vi "UDSWrapper.vi"(0 "UDS Action":T4, 1 "Session Type":u16(ring) items=["Default Session"=1, "ECU Programming Session"=2, "ECU Extended Diagnostic Session"=3], 2 "Reset Mode":u16(ring) items=["Hard Reset"=1, "Key Off On Reset"=2, "Soft Reset"=3, "Enable Rapid Power Shutdown "=4, "Disable Rapid Power Shutdown"=5], 3 "SessionID":string, 5 "UDS Session Parameters":T1={"XNET Interface"="CAN1@nixnet", "BaudRate"=500000, "Transmit ID"=470077443, "Receive ID"=470073347} {"Receive ID" format="%x"; "Transmit ID" format="%x"}, 7 "Tester Present":T3={"Start Tester Present"=FALSE, "Tester Present Period"=1.0}, 9 "ID":u16 format="%.0x", 11 "error in (no error)":errorcluster, 12 "Byte Data To Write":u8[](array[numeric]) format="%.0x", 13 "String Data To Write":string) -> (6 "Success ?":bool, 8 "Read Data":T2, 15 "error out":errorcluster)   [LabVIEW 2021, in "Lunar UDS CAN.lvlib"]
uses:
  Lunar UDS CAN.lvlib
  Controls/UDSActions.ctl
  Controls/UDSReadData.ctl
  Controls/UDSSessionParameters.ctl
  <vilib>/Automotive Diagnostic Command Set/Diagnostic Transport.llb/Diag Reference.ctl
  <vilib>/Automotive Diagnostic Command Set/Diagnostic Transport.llb/Transport Protocol Selector.ctl
  <vilib>/Automotive Diagnostic Command Set/Diagnostic Transport.llb/DoIP Protocol Version.ctl
  <vilib>/Automotive Diagnostic Command Set/Diagnostic Transport.llb/Diag Globals.ctl
  <vilib>/addons/Automotive Diagnostic Command Set/NI_Automotive Diagnostic Command Set.lvlib
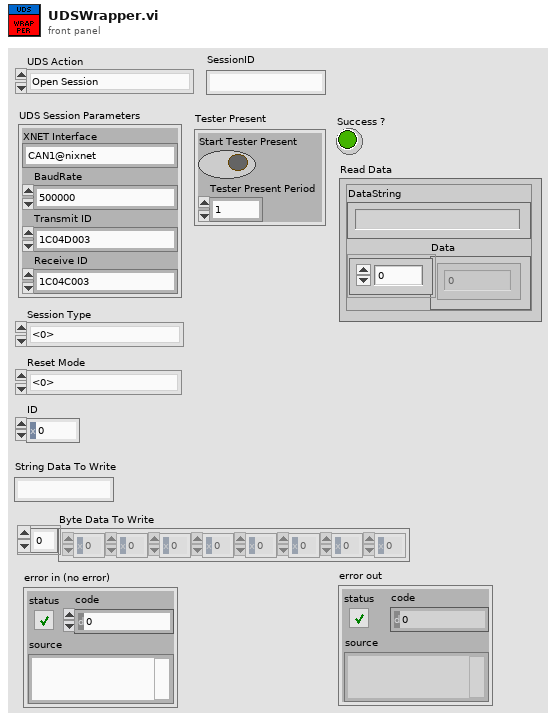
[diagram p1: front panel]
types:
  T1 = typedef "Lunar UDS CAN.lvlib/UDSSessionParameters.ctl" = cluster{"XNET Interface":string, "BaudRate":u64, "Transmit ID":i32, "Receive ID":i32}
  T2 = typedef "Lunar UDS CAN.lvlib/UDSReadData.ctl" = cluster{"DataString":string, "Data":i32[]}
  T3 = cluster{"Start Tester Present":bool, "Tester Present Period":dbl}
  T4 = typedef "Lunar UDS CAN.lvlib/UDSActions.ctl" = enum16{"Open Session", "Connect To Diagnostic Session", "Send Tester Present", "ECU Reset", "Write String Data", "Write Byte Data", "Read Data", "Close Session", "Close All Sessions"}
  T5 = typedef "NI_Automotive Diagnostic Command Set.lvlib/Diag Reference.ctl" = cluster{"Diag CAN Handle":u32, "Transport Protocol":T6, "Receive Address Extension":u8, "Transmit Address Extension":u8, "Receive CAN Id":u32, "Transmit CAN Id":u32, "Log Frames ?":bool, "My TP Address":u8, "Other TP Address":u8, "T1":u16, "T2":u16, "T3":u16, "T4":u16, "Tx SN":u8, "Block Size":u8, "Rx SN":u8, "VW TP Initialized?":bool, "Tx block no":u8, "baud rate":u64, "Interface":string, "Channel Diag CAN Handle":u32, "UDP Connection ID":refnum<k16>, "TCP Connection ID":refnum<k5>, "Target IP Addr":u32, "Source Address":u16, "Target Address":u16, "Send Header NACK?":bool, "DLL Handle":u32, "NAD":u8, "Time Stamp read first":dbl, "Time Stamp read last":dbl, "Time Stamp write first":dbl, "Time Stamp write last":dbl, "Time Stamp write":dbl, "Time Stamp read":dbl, " I/O Mode":u32, "FD Baudrate":u64, "TX_DL":u16, "RX_DL":u16, "DoIP Protocol Version":T7, " Selected I/O Mode":u32, "TesterPresent Counter":u32, "TesterPresent Limit":u32, "TesterPresent Tick[ms]":i32, "TesterPresent RequireResponse?":bool, "TesterPresent Stored Ref?":bool, "TesterPresent Message":u8[], "TesterPresent Task Handle":i32, "TesterPresent Semaphore":T8, "Response Plausibility Check":u32, "Default Version?":bool, "Diagostic Globals":T9, "Session-based Properties?":bool, "NI-XNET IP Stack Reference":i64, "NI-XNET IP Stack TCP Reference":i64, "NI-XNET IP Stack UDP Reference":i64, "NI-XNET IP Stack Local Interface":string, "Functional CAN Id":u32, "Diag CAN Queue":refnum<queue>, "Frame Fillling Mode":u32, "DoIP Acknowledge Mode":u32, "Message Buffer":u8[]}
  T6 = typedef "NI_Automotive Diagnostic Command Set.lvlib/Transport Protocol Selector.ctl" = enum16{"ISO TP - Normal Mode", "ISO TP - Mixed Mode", "VW TP 2.0", "Diagnostics on IP", "ISO TP LIN"}
  T7 = typedef "NI_Automotive Diagnostic Command Set.lvlib/DoIP Protocol Version.ctl" = u8
  T8 = typedef "Semaphore RefNum" = refnum<k1>
  T9 = typedef "NI_Automotive Diagnostic Command Set.lvlib/Diag Globals.ctl" = cluster{"Timeout FC (Bs)":u32, "Timeout CF (Cr)":u32, "Timeout Diag Command":u32, "Receive Block Size (BS)":u8, "Wait Time CF (STmin)":u8, "Max Waits (N_WFTmax)":u8, "Waits to Send (N_WAIT)":i32, "Time between Waits (TW)":u32, "Fill CAN Frames?":bool, "Fill Byte":u32, "Invalid Response as Error?":bool, "Max RspPending Count":u32, "VWTP Command Timeout":u32, "Transport Protocol":T6, "Diag CAN Handle":u32, "DLL Handle":u32, "Timeout RspPending":u32}
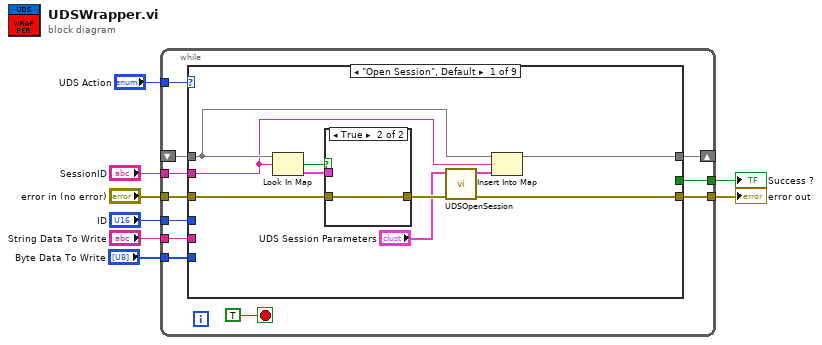
[diagram p0: block diagram]
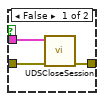
[diagram p2: hidden frame]
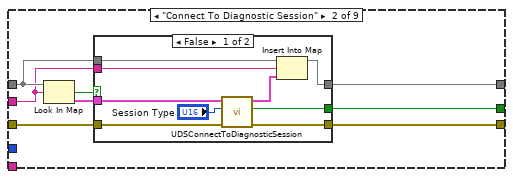
[diagram p3: hidden frame]
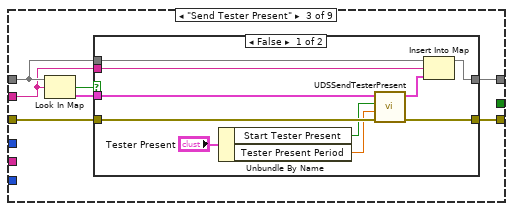
[diagram p5: hidden frame]
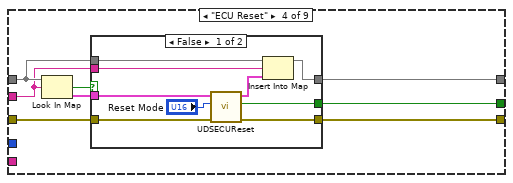
[diagram p7: hidden frame]
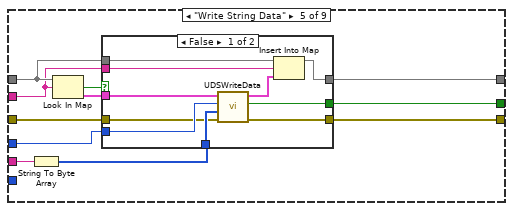
[diagram p9: hidden frame]
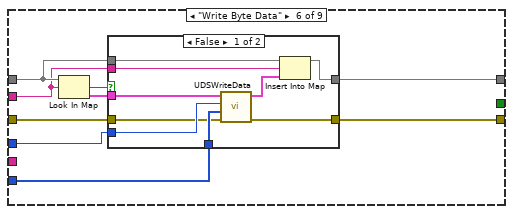
[diagram p11: hidden frame]
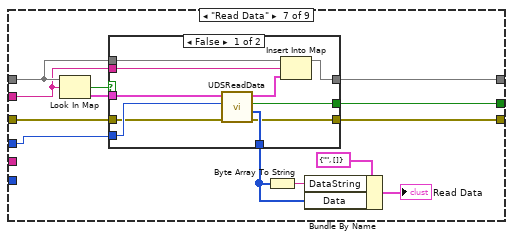
[diagram p13: hidden frame]
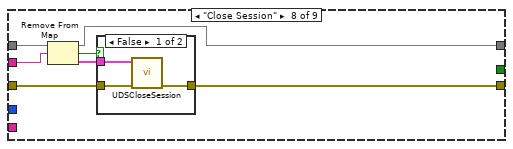
[diagram p15: hidden frame]
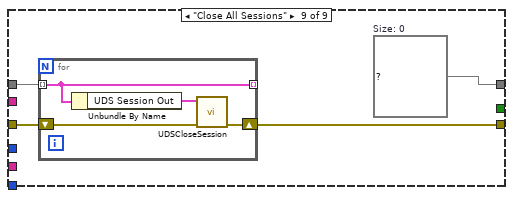
[diagram p17: hidden frame]
diagram:
  n1 = while {
    tunnel: "UDS Action" -> [w18]
    tunnel: "error in (no error)" -> [w17]
    tunnel: [w16] -> w6
    tunnel: [w15] -> w5
    tunnel: "ID" -> [w14]
    tunnel: "Byte Data To Write" -> [w13]
    tunnel: "String Data To Write" -> [w12]
    tunnel: "SessionID" -> [w11]
    shift-right: [w9] -> _
    shift-left: _ -> [w10]
    stop <- TRUE stop-if-true
    n2 = case shown="\"Open Session\", Default" w18 {
      tunnel: w17 -> [w26 w39 w57 w77 w98 w120 w140 w163 w171]
      tunnel: [w29 w38 w53 w76 w97 w119 w141 w159 w170] -> w16
      tunnel: [_ w37 _ w73 w94 _ w134 _ _] -> w15
      tunnel: w14 -> [_ _ _ _ w95 w117 w139 _ _]
      tunnel: w13 -> [_ _ _ _ _ w118 _ _ _]
      tunnel: w12 -> [_ _ _ _ w101 _ _ _ _]
      tunnel: w11 -> [w22 w35 w55 w74 w92 w114 w136 w161 _]
      tunnel: w10 -> [w24 w36 w56 w75 w93 w115 w137 w162 w172]
      tunnel: [w21 w34 w54 w72 w91 w116 w135 w160 w173] -> w9
      frame "Open Session", Default {
        n3 = Look In Map(map=w24, key=w22) -> (key not found?=w28:bool, value=w27:T5)  [unwired: 1 in]
        n4 = case shown="True" w28 {
          tunnel: w27 -> [w32 _]
          tunnel: w26 -> [w31 w33]
          tunnel: [w30 w33] -> w25
          frame False {
            n5 = call "UDSCloseSession.vi"("error in (no error)"=w31, "UDS Session In"=w32) -> ("error out"=w30:errorcluster)  [unwired: 9 in]
          }
          frame True {
          }
        }
        n6 = call "UDSOpenSession.vi"("error in (no error)"=w25, "UDS Session Parameters"="UDS Session Parameters") -> ("error out"=w29:errorcluster, "UDS Session Out"=w23:T5)  [unwired: 8 in]
        n7 = Insert Into Map(map in=w24, key=w22, value=w23) -> (map out=w21:map{string, T5})  [unwired: 2 out]
      }
      frame "Connect To Diagnostic Session" {
        n8 = Look In Map(map=w36, key=w35) -> (key not found?=w41:bool, value=w40:T5)  [unwired: 1 in]
        n9 = case shown="False" w41 {
          tunnel: w40 -> [w47 _]
          tunnel: w39 -> [w50 w52]
          tunnel: [w49 w52] -> w38
          tunnel: [w48 _] -> w37
          tunnel: w36 -> [w44 w51]
          tunnel: w35 -> [w43 _]
          tunnel: [w42 w51] -> w34
          frame False {
            n10 = call "UDSConnectToDiagnosticSession.vi"("error in (no error)"=w50, "Session Type"="Session Type", "UDS Session In"=w47) -> ("error out"=w49:errorcluster, "Connection Success ?"=w48:bool, "UDS Session Out"=w45:T5)  [unwired: 6 in]
            n11 = Insert Into Map(map in=w44, key=w43, value=w45) -> (map out=w42:map{string, T5})  [unwired: 2 out]
          }
          frame True {
          }
        }
      }
      frame "Send Tester Present" {
        n12 = Look In Map(map=w56, key=w55) -> (key not found?=w59:bool, value=w58:T5)  [unwired: 1 in]
        n13 = case shown="False" w59 {
          tunnel: w58 -> [w62 _]
          tunnel: w57 -> [w64 w71]
          tunnel: [w65 w71] -> w53
          tunnel: w56 -> [w69 w70]
          tunnel: w55 -> [w68 _]
          tunnel: [w67 w70] -> w54
          frame False {
            n14 = Unbundle By Name("Tester Present") -> ("Start Tester Present"=w61:bool, "Tester Present Period"=w60:dbl)
            n15 = call "UDSSendTesterPresent.vi"("error in (no error)"=w64, "Period"=w60, "Start"=w61, "UDS Session In"=w62) -> ("error out"=w65:errorcluster, "UDS Session Out"=w66:T5)  [unwired: 6 in]
            n16 = Insert Into Map(map in=w69, key=w68, value=w66) -> (map out=w67:map{string, T5})  [unwired: 2 out]
          }
          frame True {
          }
        }
      }
      frame "ECU Reset" {
        n17 = Look In Map(map=w75, key=w74) -> (key not found?=w79:bool, value=w78:T5)  [unwired: 1 in]
        n18 = case shown="False" w79 {
          tunnel: w78 -> [w88 _]
          tunnel: w77 -> [w87 w90]
          tunnel: [w85 w90] -> w76
          tunnel: w75 -> [w83 w89]
          tunnel: w74 -> [w82 _]
          tunnel: [w81 _] -> w73
          tunnel: [w80 w89] -> w72
          frame False {
            n19 = call "UDSECUReset.vi"("error in (no error)"=w87, "Reset Mode"="Reset Mode", "UDS Session In"=w88) -> ("error out"=w85:errorcluster, "success?"=w81:bool, "UDS Session Out"=w84:T5)  [unwired: 6 in]
            n20 = Insert Into Map(map in=w83, key=w82, value=w84) -> (map out=w80:map{string, T5})  [unwired: 2 out]
          }
          frame True {
          }
        }
      }
      frame "Write String Data" {
        n21 = String To Byte Array(string=w101) -> (unsigned byte array=w96:u8[])
        n22 = Look In Map(map=w93, key=w92) -> (key not found?=w100:bool, value=w99:T5)  [unwired: 1 in]
        n23 = case shown="False" w100 {
          tunnel: w99 -> [w102 _]
          tunnel: w98 -> [w105 w113]
          tunnel: [w106 w113] -> w97
          tunnel: w93 -> [w111 w112]
          tunnel: w92 -> [w110 _]
          tunnel: [w109 w112] -> w91
          tunnel: w96 -> [w108 _]
          tunnel: w95 -> [w107 _]
          tunnel: [w104 _] -> w94
          frame False {
            n24 = call "UDSWriteData.vi"("error in (no error)"=w105, "Data To Write"=w108, "ID"=w107, "UDS Session In"=w102) -> ("error out"=w106:errorcluster, "success?"=w104:bool, "UDS Session Out"=w103:T5)  [unwired: 5 in]
            n25 = Insert Into Map(map in=w111, key=w110, value=w103) -> (map out=w109:map{string, T5})  [unwired: 2 out]
          }
          frame True {
          }
        }
      }
      frame "Write Byte Data" {
        n26 = Look In Map(map=w115, key=w114) -> (key not found?=w122:bool, value=w121:T5)  [unwired: 1 in]
        n27 = case shown="False" w122 {
          tunnel: w121 -> [w123 _]
          tunnel: w120 -> [w126 w133]
          tunnel: [w125 w133] -> w119
          tunnel: w115 -> [w131 w132]
          tunnel: w114 -> [w130 _]
          tunnel: [w129 w132] -> w116
          tunnel: w118 -> [w128 _]
          tunnel: w117 -> [w127 _]
          frame False {
            n28 = call "UDSWriteData.vi"("error in (no error)"=w126, "Data To Write"=w128, "ID"=w127, "UDS Session In"=w123) -> ("error out"=w125:errorcluster, "UDS Session Out"=w124:T5)  [unwired: 5 in, 1 out]
            n29 = Insert Into Map(map in=w131, key=w130, value=w124) -> (map out=w129:map{string, T5})  [unwired: 2 out]
          }
          frame True {
          }
        }
      }
      frame "Read Data" {
        n30 = Look In Map(map=w137, key=w136) -> (key not found?=w143:bool, value=w142:T5)  [unwired: 1 in]
        n31 = case shown="False" w143 {
          tunnel: w142 -> [w149 _]
          tunnel: w140 -> [w150 w158]
          tunnel: [w151 w158] -> w141
          tunnel: w137 -> [w156 w157]
          tunnel: w136 -> [w155 _]
          tunnel: [w154 w157] -> w135
          tunnel: w139 -> [w153 _]
          tunnel: [w152 _] -> w138
          tunnel: [w148 _] -> w134
          frame False {
            n32 = call "UDSReadData.vi"("error in (no error)"=w150, "ID"=w153, "UDS Session In"=w149) -> ("error out"=w151:errorcluster, "data out"=w152:u8[], "success?"=w148:bool, "UDS Session Out"=w147:T5)  [unwired: 5 in]
            n33 = Insert Into Map(map in=w156, key=w155, value=w147) -> (map out=w154:map{string, T5})  [unwired: 2 out]
          }
          frame True {
          }
        }
        n34 = Byte Array To String(unsigned byte array=w138) -> (string=w146:string)
        n35 = Bundle By Name(cluster=cluster{"DataString":string, "Data":u8[]} {"DataString"="", "Data"=[]} ("input cluster"), "DataString"=w146, "Data"=w138) -> (→"Read Data":cluster{"DataString":string, "Data":u8[]})
      }
      frame "Close Session" {
        n36 = Remove From Map(10:w161, 11:w162) -> (1:w164:T5, 2:w165:bool, 3:w160:map{string, T5})
        n37 = case shown="False" w165 {
          tunnel: w164 -> [w168 _]
          tunnel: w163 -> [w167 w169]
          tunnel: [w166 w169] -> w159
          frame False {
            n38 = call "UDSCloseSession.vi"("error in (no error)"=w167, "UDS Session In"=w168) -> ("error out"=w166:errorcluster)  [unwired: 9 in]
          }
          frame True {
          }
        }
      }
      frame "Close All Sessions" {
        w173 = map{string, T5} {}  # Size: 0
        n39 = for {
          tunnel: [w176] -> _ mode=indexing
          tunnel: w172 -> [w176] mode=indexing
          shift-right: [w174] -> w170
          shift-left: w171 -> [w177]
          n40 = Unbundle By Name(w176) -> ("UDS Session Out"=w175:T5)
          n41 = call "UDSCloseSession.vi"("error in (no error)"=w177, "UDS Session In"=w175) -> ("error out"=w174:errorcluster)  [unwired: 9 in]
        }
      }
    }
  }
  "error out" <- w6
  "Success ?" <- w5
